vi "JoyTest.vi"() -> ()   [LabVIEW 2016]
uses:
  <vilib>/Rock Robotics/WPI/Joystick/WPI_JoystickDevRef.ctl
  <vilib>/Rock Robotics/WPI/Joystick/WPI_JoystickDeviceEnum.ctl
  <vilib>/Rock Robotics/WPI/Utilities/WPI_GetSetVariantRefNum.vi
  <vilib>/Rock Robotics/WPI/RobotDrive/WPI_RobotDriveArcadeDrive_Standard(NoSaturation).vi
panel:
  out "POVs":i16[](array[numeric])
  out "Buttons":bool[](array[boolean])
  out "Axes":dbl[](array[numeric])
  out "JoystickDevRef":T1
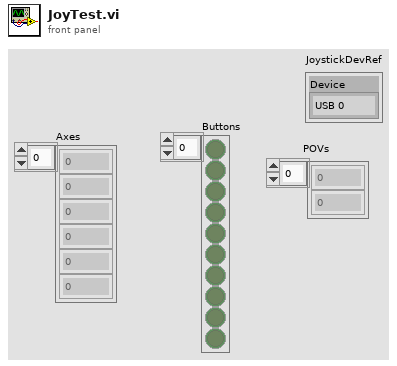
[diagram p1: front panel]
types:
  T1 = typedef "WPI_JoystickDevRef.ctl" = cluster{"Device":T2}
  T2 = typedef "WPI_JoystickDeviceEnum.ctl" = enum16{"USB 0", "USB 1", "USB 2", "USB 3", "USB 4", "USB 5"}
  T3 = typedef "WPI_RobotDriveDevRef.ctl" = cluster{"DevStatus":errorcluster, "Motors[]":T4[], "Square Inputs":bool, "Max Output":dbl}
  T4 = typedef "WPI_MotorControlDeviceRef.ctl" = cluster{"DeviceStatus":errorcluster, "Type":T5, "PWM":cluster{"PWM Channel":T6, "DeadBand":T7}, "CAN":cluster{"Device Number":u8, "SetOutput VI Ref":variant, "GetOutput VI Ref":variant, "Enable VI Ref":variant, "Disable VI Ref":variant, "Data":variant}, "Invert":bool}
  T5 = typedef "WPI_MotorControlType.ctl" = enum16{"PWM", "CAN"}
  T6 = typedef "FPGA_DIOPWMChannel.ctl" = enum8{"PWM 0", "PWM 1", "PWM 2", "PWM 3", "PWM 4", "PWM 5", "PWM 6", "PWM 7", "PWM 8", "PWM 9", "PWM MXP 0", "PWM MXP 1", "PWM MXP 2", "PWM MXP 3", "PWM MXP 4", "PWM MXP 5", "PWM MXP 6", "PWM MXP 7", "PWM MXP 8", "PWM MXP 9", "Invalid"}
  T7 = typedef "WPI_PWMDeadband.ctl" = cluster{"Name":string, "maxPositivePwm":i32, "minPositivePwm":i32, "centerPwm":i32, "maxNegativePwm":i32, "minNegativePwm":i32, "angularRange":u16}
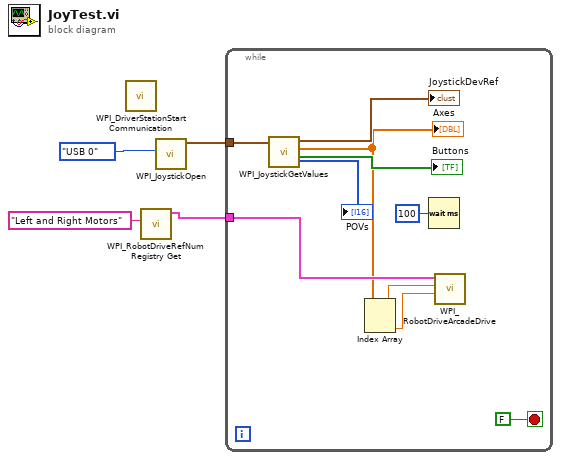
[diagram p0: block diagram]
diagram:
  n1 = call <vilib>:"WPI_DriverStationStart Communication.vi"() -> ()  [unwired: 12 in]
  n2 = call <vilib>:"WPI_RobotDriveRefNum Registry Get.vi"("refnum name"="Left and Right Motors") -> ("RobotDriveDevRef"=w2:T3)  [unwired: 9 in, 1 out]
  n3 = call <vilib>:"WPI_JoystickOpen.vi"("JoystickDevice"=WPI_JoystickDeviceEnum."USB 0") -> ("JoystickDevRef"=w3:T1)  [unwired: 10 in]
  n4 = while {
    tunnel: w3 -> [w13]
    tunnel: w2 -> [w8]
    stop <- FALSE stop-if-true
    n5 = call <vilib>:"WPI_JoystickGetValues.vi"("JoystickDevRef"=w13) -> ("Buttons"=→"Buttons":bool[], "Axes"=w7:dbl[], "JoystickDevRef"=→"JoystickDevRef":T1, "POVs"=→"POVs":i16[])  [unwired: 6 in, 1 out]
    "Axes" <- w7
    n6 = Index Array(array=w7) -> (element #1=w6:dbl, element #2=w5:dbl)  [unwired: 2 in]
    n7 = Wait (ms)(milliseconds to wait=u32 100) -> ()  [unwired: 1 out]
    n8 = call-poly <vilib>:"WPI_RobotDriveArcadeDrive.vi"("Y axis value"=w5, "X axis value"=w6, "RobotDriveDevRef"=w8) -> ()  [unwired: 6 in, 3 out]
  }
